vi "DDS - Triangle.vi"(7 "Reset Accumulator":bool, 10 "Accumulator Increment":fxp<+,32,32>) -> (1 "Accumulator Value":fxp<+,32,32>, 2 "data out":i16 caption="Sine Data Out")   [LabVIEW 2015]
uses:
  <vilib>/rvi/FXPMathLib/FxpAdd/XNode/nifxpmath_Add.xnode
  <vilib>/rvi/FXPMathLib/sim/FxpSim.dll
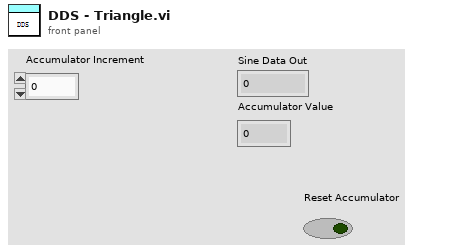
[diagram p1: front panel]
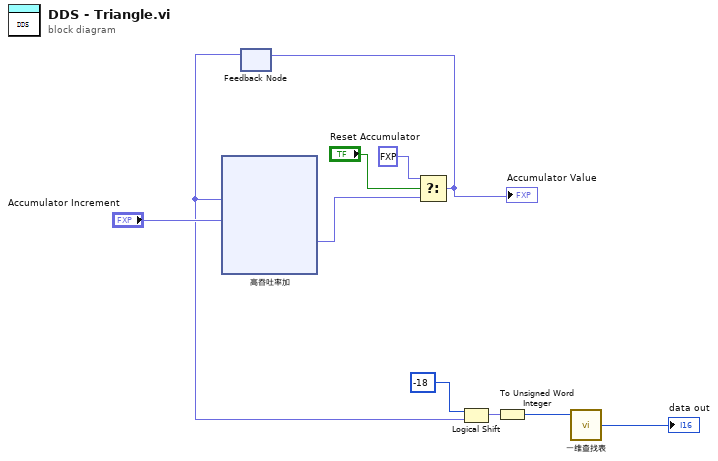
[diagram p0: block diagram]
diagram:
  n1 = feedback #1() -> (w1:fxp<+,32,32>)  [unwired: 1 in]
  n2 = xnode ("高吞吐率加")("x"=w1, "y"="Accumulator Increment") -> ("x+y"=w8:fxp<+,32,32>)  [unwired: 1 out]
  n3 = Select(t=fxp<+,32,32> 0.0, s="Reset Accumulator", f=w8) -> (s? t:f=w9:fxp<+,32,32>)
  "Accumulator Value" <- w9
  n4 = feedback-in #1(w9) -> ()
  n5 = Logical Shift(y=i16 -18, x=w1) -> (x << y=w3:fxp<+,32,32>)
  n6 = To Unsigned Word Integer(number=w3) -> (unsigned 16bit integer=w2:u16)
  n7 = call "一维查找表"("address"=w2) -> ("data out"=→"data out":i16)  [unwired: 8 in]
